vi "Async or Show Example.vi"() -> ()   [LabVIEW 2015]
uses:
  SubVIs/UI.vi
  <vilib>/Erdos Miller/LV-Async/async-or-show-xnode/LV-Async-Or-Show.xnode
panel:
  in  "Numeric Control":dbl
  in  "Launch":bool
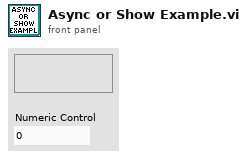
[diagram p1: front panel]
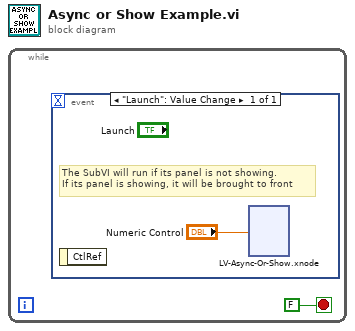
[diagram p0: block diagram]
diagram:
  n1 = while {
    stop <- FALSE stop-if-true
    n2 = event shown="[0] \"Launch\": Value Change" {
      selector: _ -> [_]
      dyn-events: _ -> [_]
      timeout: _ -> [_]
      event "Launch": Value Change {
        # "The SubVI will run if its panel is not showing.\nIf its panel is showing, it will be brought to front"
        n3 = event-data() -> ()  [unwired: 1 in, 1 out]
        n4 = xnode "LV-Async-Or-Show.xnode"("Numeric Control"="Numeric Control") -> ()  [unwired: 1 in, 1 out]
      }
    }
  }
